vi "Read Queue.vi"(11 "BluePlotHandle in":refnum<class "BluePlotHandle.lvclass">) -> (1 "Valid?":bool, 2 "Queue":refnum<queue>, 3 "BluePlotHandle out":refnum<class "BluePlotHandle.lvclass">)   [LabVIEW 2021, in "BluePlot.lvlib" / "BluePlotHandle.lvclass"]
uses:
  BluePlotHandle.lvclass
  TypeDefs/plot handle queue data.ctl
  TypeDefs/Plot QSM action.ctl
  BluePlotHandle.lvclass/BluePlotHandle.ctl
  BluePlot.lvlib
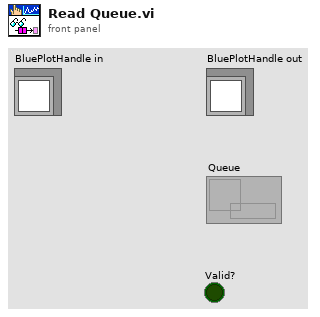
[diagram p1: front panel]
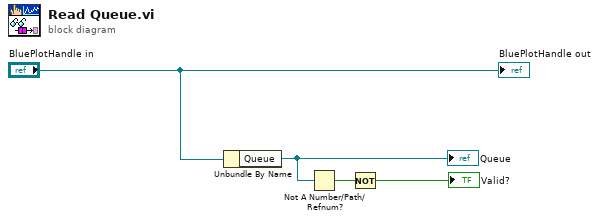
[diagram p0: block diagram]
diagram:
  n1 = Unbundle By Name("BluePlotHandle in") -> ("Queue"=w1:refnum<queue>)
  "Queue" <- w1
  n2 = Not A Number/Path/Refnum?(number/path/refnum=w1) -> (NaN/Path/Refnum?=w4:bool)
  n3 = Not(x=w4) -> (.not. x?=→"Valid?":bool)
  "BluePlotHandle out" <- "BluePlotHandle in"
